vi "Server_Login.vi"(7 "connection ID":refnum<k5>, 8 "error in":errorcluster, 11 "User Name":string) -> (0 "error out":errorcluster, 3 "User Data":T1={"Name"="Guset", "Email"="", "Phone Number"="", "User Picture"=array225x225[50625 elements], "Last Login Time"=timestamp(0 s since 1904-01-01)})   [LabVIEW 2018, in "Cloud Server.lvlib"]
uses:
  Cloud Server.lvlib
  Com VIs/Data Def/User Data.ctl
  Data Def/Server_Connection Manager Method.ctl
  Data Def/Server_Connection Properties.ctl
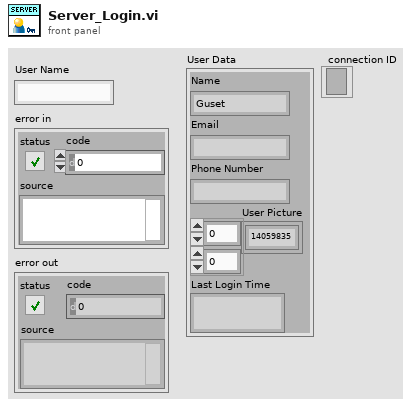
[diagram p1: front panel]
types:
  T1 = typedef "User Data.ctl" = cluster{"Name":string, "Email":string, "Phone Number":string, "User Picture":u32[][], "Last Login Time":timestamp}
  T2 = typedef "Cloud Server.lvlib/Server_Connection Manager Method.ctl" = enum16{"Initialize", "Add", "Get", "Set Properties", "Get Properties", "Close", "Release"}
  T3 = typedef "Cloud Server.lvlib/Server_Connection Properties.ctl" = cluster{"User Data":T1, "Data":waveform(dbl)}
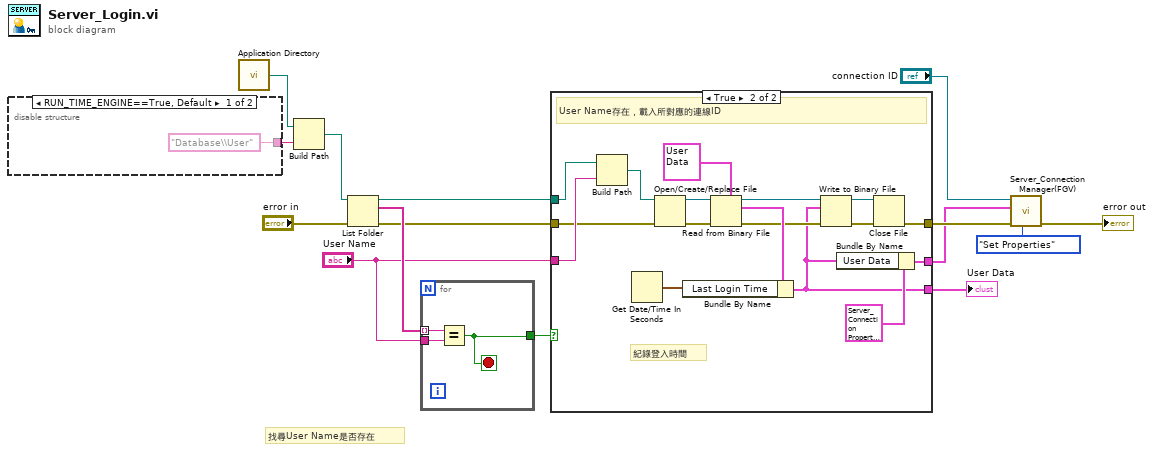
[diagram p0: block diagram]
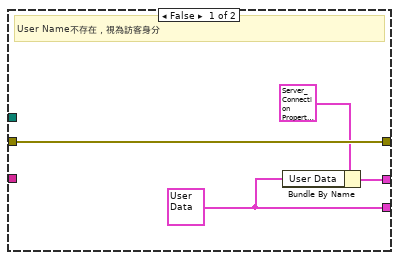
[diagram p2: hidden frame]
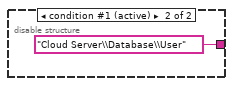
[diagram p3: hidden frame]
diagram:
  # "找尋User Name是否存在"
  n1 = disable-structure shown="RUN_TIME_ENGINE==True, Default" {
    disable-tunnel: ["Database\\User" ("name or relative path") "Cloud Server\\Database\\User" ("name or relative path")] -> w15
    frame condition #0 {
    }
    frame condition #1 (active) {
    }
  }
  n2 = call <vilib>:"Application Directory.vi"() -> ("Application Directory"=w14:path)
  n3 = Build Path(base path=w14, name or relative path=w15) -> (appended path=w12:path)
  n4 = List Folder(path=w12, error in="error in") -> (path out=w8:path, filenames=w11:string[], error out=w9:errorcluster)  [unwired: 2 in, 1 out]
  n5 = for {
    tunnel: "User Name" -> [w20]
    tunnel: [w19] -> w10
    tunnel: w11 -> [w18] mode=indexing
    stop <- w19 stop-if-true
    n6 = Equal?(x=w18, y=w20) -> (x = y?=w19:bool)
  }
  n7 = case shown="True" w10 {
    tunnel: w9 -> [w24 w39]
    tunnel: w8 -> [_ w41]
    tunnel: "User Name" -> [_ w40]
    tunnel: [w22 w27] -> w6
    tunnel: [w24 w26] -> w4
    tunnel: [w21 w25] -> w3
    frame False {
      w22 = T1 {"Name"="Guest", "Email"="", "Phone Number"="", "User Picture"=array225x225[50625 elements], "Last Login Time"=timestamp(0 s since 1904-01-01)} ("Array")
      # "User Name不存在，視為訪客身分"
      n8 = Bundle By Name(cluster=T3 {"User Data"={"Name"="", "Email"="", "Phone Number"="", "User Picture"=array225x225[50625 elements], "Last Login Time"=timestamp(0 s since 1904-01-01)}, "Data"={"t0"=timestamp(0 s since 1904-01-01), "dt"=1.0, "Y"=[]}} ("Connection Properties In"), "User Data"=w22) -> (w21:T3)
    }
    frame True {
      # "紀錄登入時間"
      # "User Name存在，載入所對應的連線ID"
      n9 = Build Path(base path=w41, name or relative path=w40) -> (appended path=w38:path)
      n10 = Get Date/Time In Seconds() -> (seconds since 1Jan1904=w32:timestamp)
      n11 = Open/Create/Replace File(file path (use dialog)=w38, error in=w39) -> (refnum out=w36:refnum<file>, error out=w37:errorcluster)  [unwired: 4 in, 1 out]
      n12 = Read from Binary File(5:T1 {"Name"="Guset", "Email"="", "Phone Number"="", "User Picture"=array225x225[50625 elements], "Last Login Time"=timestamp(0 s since 1904-01-01)} ("Array"), 8:w37, 11:w36) -> (0:w31:errorcluster, 2:w33:T1, 3:w30:refnum<file>)  [unwired: 3 in, 1 out]
      n13 = Bundle By Name(cluster=w33, "Last Login Time"=w32) -> (w27:T1)
      n14 = Write to Binary File(file (use dialog)=w30, data=w27, error in=w31) -> (refnum out=w29:refnum<file>, error out=w28:errorcluster)  [unwired: 3 in, 1 out]
      n15 = Bundle By Name(cluster=T3 {"User Data"={"Name"="", "Email"="", "Phone Number"="", "User Picture"=array225x225[50625 elements], "Last Login Time"=timestamp(0 s since 1904-01-01)}, "Data"={"t0"=timestamp(0 s since 1904-01-01), "dt"=1.0, "Y"=[]}} ("Connection Properties In"), "User Data"=w27) -> (w25:T3)
      n16 = Close File(refnum=w29, error in=w28) -> (error out=w26:errorcluster)  [unwired: 1 out]
    }
  }
  "User Data" <- w6
  n17 = call "Server_Connection Manager(FGV).vi"("Connection Manager Method(Get)"=Server_Connection_Manager_Method."Set Properties", "error in"=w4, "Connection Properties In"=w3, "Connection In"="connection ID") -> ("error out"=→"error out":errorcluster)  [unwired: 3 in, 4 out]
